vi "Pre Launch Init.vi"(11 "Phoenix in":refnum<class "Phoenix.lvclass">) -> (0 "error out":errorcluster, 3 "Phoenix out":refnum<class "Phoenix.lvclass">)   [LabVIEW 2022 SP3, in "Phoenix.lvlib" / "Phoenix.lvclass"]
doc: "(<B>Filename</B>: Actor Framework.lvlib:Actor.lvclass:Pre Launch Init.vi)\n\nDefines behavior that occurs after the Launch Actor method is invoked but before the actor's Actor Core method begins running.\n\nThe Pre Launch Init method is guaranteed to finish before the Launch Actor method returns to its caller and before the actor itself receives any messages. Any references that the Pre Launch Init method obtains are guaranteed to have the same lifetime as the actor itself. Any errors that the Pre Launch Init method returns will abort the launch.\n\nBy default, this method does nothing. A descendant class may override it to define behavior."
uses:
  Phoenix.lvclass
  <vilib>/MGI/Monitored Actor/Monitored Actor/Monitored Actor/Monitored Actor.lvclass
  Phoenix.lvclass/Phoenix.ctl
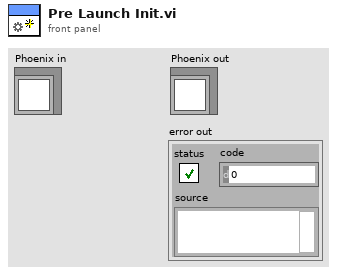
[diagram p1: front panel]
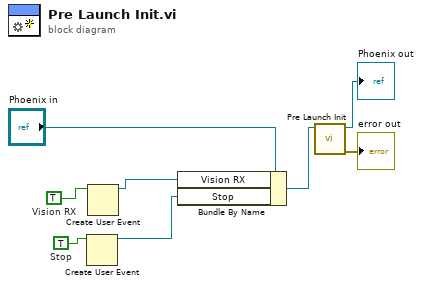
[diagram p0: block diagram]
diagram:
  w1 = TRUE  # Vision RX
  w2 = TRUE  # Stop
  n1 = Create User Event(user event datatype=w2) -> (user event=w3:refnum<user-event>)  [unwired: 1 in, 1 out]
  n2 = Create User Event(user event datatype=w1) -> (user event=w4:refnum<user-event>)  [unwired: 1 in, 1 out]
  n3 = Bundle By Name(cluster="Phoenix in", "Vision RX"=w4, "Stop"=w3) -> (w5:refnum<class "Phoenix.lvclass">)
  n4 = call-parent "Pre Launch Init.vi"("Monitored Actor in"=w5) -> ("error out"=→"error out":errorcluster, "Monitored Actor out"=→"Phoenix out":refnum<class "Phoenix.lvclass">)  [unwired: 9 in]
